vi "SRV_Write Motors Config File.vi"(0 "Motors Config File Path":path, 7 "Motor Control Config":T1[](array[typedef]) {"Release Cmds"."Motor Control Commands Array"."Value" format="%02x"; "Release Cmds"."Motor Control Commands Array"."Register" format="%02x"; "Release Cmds"."Motor Control Commands Array"."I2C Address" format="%02x"; "Press Cmds"."Motor Control Commands Array"."Value" format="%02x"; "Press Cmds"."Motor Control Commands Array"."Register" format="%02x"; "Press Cmds"."Motor Control Commands Array"."I2C Address" format="%02x"}, 11 "error in (no error)":errorcluster) -> (15 "error out":errorcluster)   [LabVIEW 2014]
doc: "Author: Mike Schultz (LogicPD, Inc)"
uses:
  SRV_Motor Control Button Config.ctl
  SRV_Motor Legos-Servo.ctl
  SRV_Motor Control Commands Cluster.ctl
  SRV_Motor Control Command Config.ctl
  SRV_Motor Control Button Icons_FALSE.ctl
  <vilib>/Utility/xml.llb/Write to XML File(string).vi
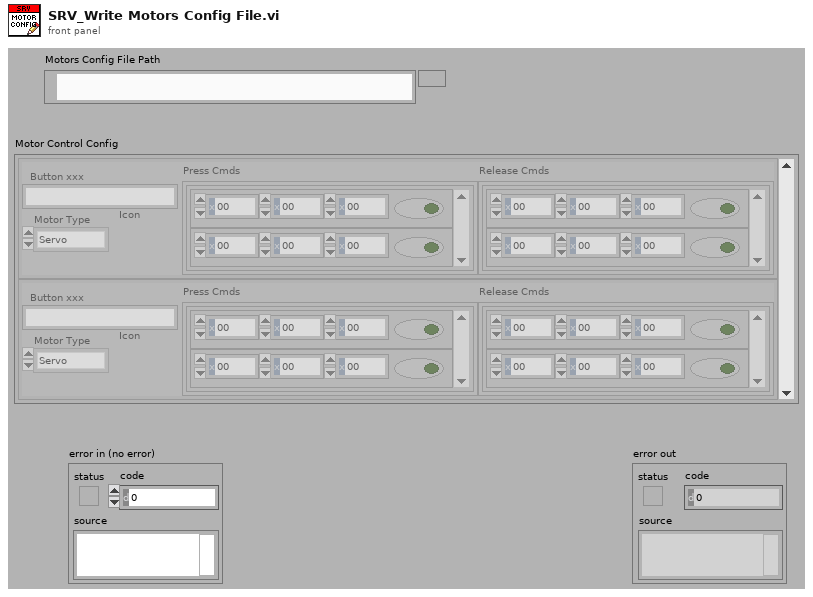
[diagram p1: front panel]
types:
  T1 = typedef "SRV_Motor Control Button Config.ctl" = cluster{"Button Name":string, "Button Label":string, "Motor Type":T2, "Press Cmds":T3, "Release Cmds":T3, "Icon":T5}
  T2 = typedef "SRV_Motor Legos-Servo.ctl" = enum16{"Servo", "Legos", "Shared Var"}
  T3 = typedef "SRV_Motor Control Commands Cluster.ctl" = cluster{"Motor Control Commands Array":T4[]}
  T4 = typedef "SRV_Motor Control Command Config.ctl" = cluster{"I2C Address":u8, "Register":u8, "Value":u8, "Active":bool}
  T5 = typedef "SRV_Motor Control Button Icons_FALSE.ctl" = u16
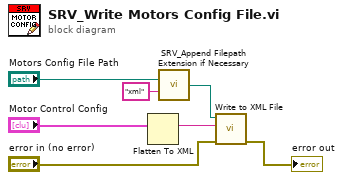
[diagram p0: block diagram]
diagram:
  n1 = Flatten To XML(anything="Motor Control Config") -> (xml string=w7:string)
  n2 = call "SRV_Append Filepath Extension if Necessary.vi"("Filepath"="Motors Config File Path", "Extension"="xml") -> ("Filepath with Extension"=w5:path)  [unwired: 13 in]
  n3 = call-poly <vilib>:"Write to XML File.vi"("error in (no error)"="error in (no error)", "XML Input"=w7, "XML File Path"=w5) -> ("error out"=→"error out":errorcluster)  [unwired: 6 in, 2 out]
